vi "ke37xx Forbidden Channels.vi"(0 "VISA Resource Name":refnum<visa-resource-name>, 1 "Channel List":string, 7 "Operation (0: Setl)":enum16{"Set", "Get", "Clear"}(ring), 11 "error in (no error)":errorcluster, 12 "Bytes To Read (1024)":u32=1024) -> (4 "VISA Resource Name Out":refnum<visa-resource-name>, 8 "Forbidden Channel List":string, 15 "error out":errorcluster)   [LabVIEW 2009, in "Keithley 3700 Series.lvlib"]
doc: "This VI allows you to set, query, or clear the list of channels that are forbidden to be closed."
uses:
  <instrlib>/Keithley 3706/Keithley 3700 Series.lvlib
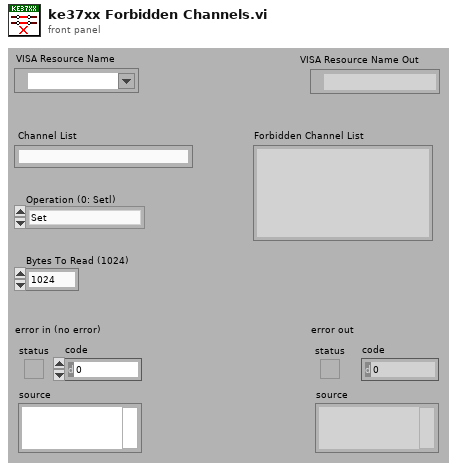
[diagram p1: front panel]
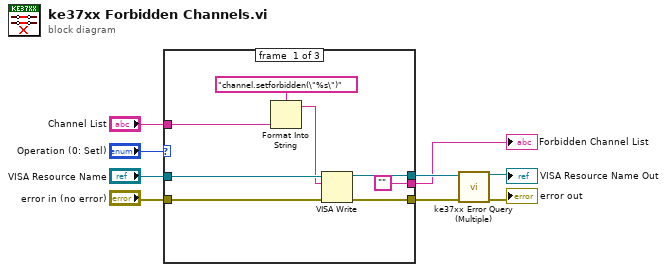
[diagram p0: block diagram]
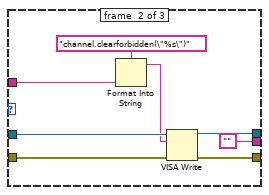
[diagram p2: hidden frame]
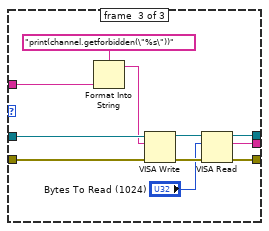
[diagram p3: hidden frame]
diagram:
  n1 = case shown="\"Set\", Default" "Operation (0: Setl)" {
    tunnel: "VISA Resource Name" -> [w17 w25 w36]
    tunnel: "error in (no error)" -> [w16 w24 w35]
    tunnel: [w15 w23 w33] -> w5
    tunnel: [w14 w22 w31] -> w4
    tunnel: ["" "" w29] -> w3
    tunnel: "Channel List" -> [w11 w19 w26]
    frame #0 {
      n2 = Format Into String(format string="channel.setforbidden(\"%s\")", w11) -> (resulting string=w12:string)  [unwired: 2 in, 1 out]
      n3 = VISA Write(VISA resource name=w17, write buffer=w12, error in (no error)=w16) -> (VISA resource name out=w15:refnum<visa-resource-name>, error out=w14:errorcluster)  [unwired: 1 out]
    }
    frame #1 {
      n4 = Format Into String(format string="channel.clearforbidden(\"%s\")", w19) -> (resulting string=w20:string)  [unwired: 2 in, 1 out]
      n5 = VISA Write(VISA resource name=w25, write buffer=w20, error in (no error)=w24) -> (VISA resource name out=w23:refnum<visa-resource-name>, error out=w22:errorcluster)  [unwired: 1 out]
    }
    frame #2 {
      n6 = Format Into String(format string="print(channel.getforbidden(\"%s\"))", w26) -> (resulting string=w27:string)  [unwired: 2 in, 1 out]
      n7 = VISA Write(VISA resource name=w36, write buffer=w27, error in (no error)=w35) -> (VISA resource name out=w34:refnum<visa-resource-name>, error out=w32:errorcluster)  [unwired: 1 out]
      n8 = VISA Read(VISA resource name=w34, byte count="Bytes To Read (1024)", error in (no error)=w32) -> (VISA resource name out=w33:refnum<visa-resource-name>, read buffer=w29:string, error out=w31:errorcluster)  [unwired: 1 out]
    }
  }
  "Forbidden Channel List" <- w3
  n9 = call <instrlib>:"ke37xx Error Query (Multiple).vi"("VISA resource name"=w5, "error in (no error)"=w4) -> ("VISA resource name out"=→"VISA Resource Name Out":refnum<visa-resource-name>, "error out"=→"error out":errorcluster)  [unwired: 12 out]
